vi "Loop Async.vi"(11 "RemoteDataService in":refnum<class "RemoteDataService.lvclass">) -> ()   [LabVIEW 2020, in "Vecto.lvlib" / "RemoteDataService.lvclass"]
uses:
  RemoteDataService.lvclass
  RemoteDataService.lvclass/RemoteDataService.ctl
  Packet.ctl
  lv-protoc/LV-Proto/Message/Message.lvclass
  Vecto.lvlib
  GroupNamesValue/GroupNamesValue.lvclass
  lv-promises/Promises/Promise/Promise.lvclass
  Group Data Type.ctl
  VectoConfig/VectoConfig.lvlib
  Publish Group Data.ctl
  EventLoggingService/EventLoggingService.lvclass
panel:
  out "Proc":i32(graph)
  out "Chart":i32(graph)
  out "Local Port":u16
  out "Bind Port":u16
  out "Bind Address":u32
  out "Node ID":u32
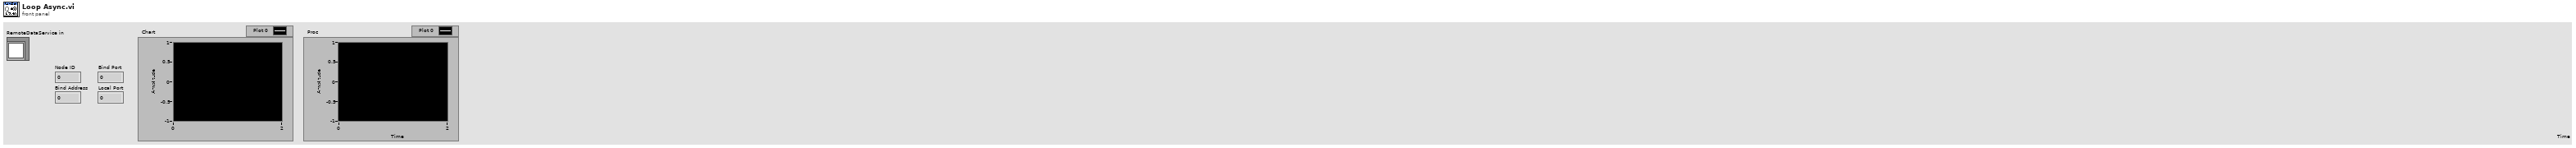
[diagram p1: front panel]
types:
  T1 = typedef "Vecto.lvlib/RemoteDataService.lvclass/Packet.ctl" = cluster{"UDP":refnum<k16>, "IP":u32, "Port":u16, "Message":refnum<class "Message.lvclass">, "Data Type":T2}
  T2 = typedef "VectoConfig.lvlib/Group Data Type.ctl" = enum16{"Double", "String", "Bool"}
  T3 = typedef "Vecto.lvlib/RemoteDataService.lvclass/Loop Data.ctl" = cluster{"Group Map":map{string, T4}, "UDP":refnum<k16>, "SequenceCountService":refnum<class "SequenceCountService.lvclass">, "Node ID":u32, "Bind Address":u32, "Bind Port":u16, "Local Port":u16, "TX Q":refnum<queue>, "Subscriptions":map{T5, T6}, "ChannelService":refnum<class "ChannelService.lvclass">, "Telemetry Config":T7}
  T4 = typedef "Vecto.lvlib/RemoteDataService.lvclass/Published Group.ctl" = cluster{"Last Publish":dbl, "Publish Address":u32, "Publish Port":u16}
  T5 = typedef "Vecto.lvlib/RemoteDataService.lvclass/Subscription.ctl" = cluster{"Multicast Address":string, "Multicast Port":u16}
  T6 = typedef "Vecto.lvlib/RemoteDataService.lvclass/Subscription Info.ctl" = cluster{"Close":refnum<user-event>, "New Data Handler":refnum<user-event>}
  T7 = typedef "VectoConfig.lvlib/Telemetry Config.ctl" = cluster{"Routing":T8, "Endpoint":T9}
  T8 = typedef "VectoConfig.lvlib/Telemetry Routing.ctl" = enum16{"Multicast", "Unicast"}
  T9 = typedef "VectoConfig.lvlib/Endpoint.ctl" = cluster{"Address":string, "Port":u16}
  T10 = typedef "Vecto.lvlib/RemoteDataService.lvclass/Publish Group Data.ctl" = cluster{"Data Msg":refnum<class "Message.lvclass">, "Group Name":string, "Data Type":T2}
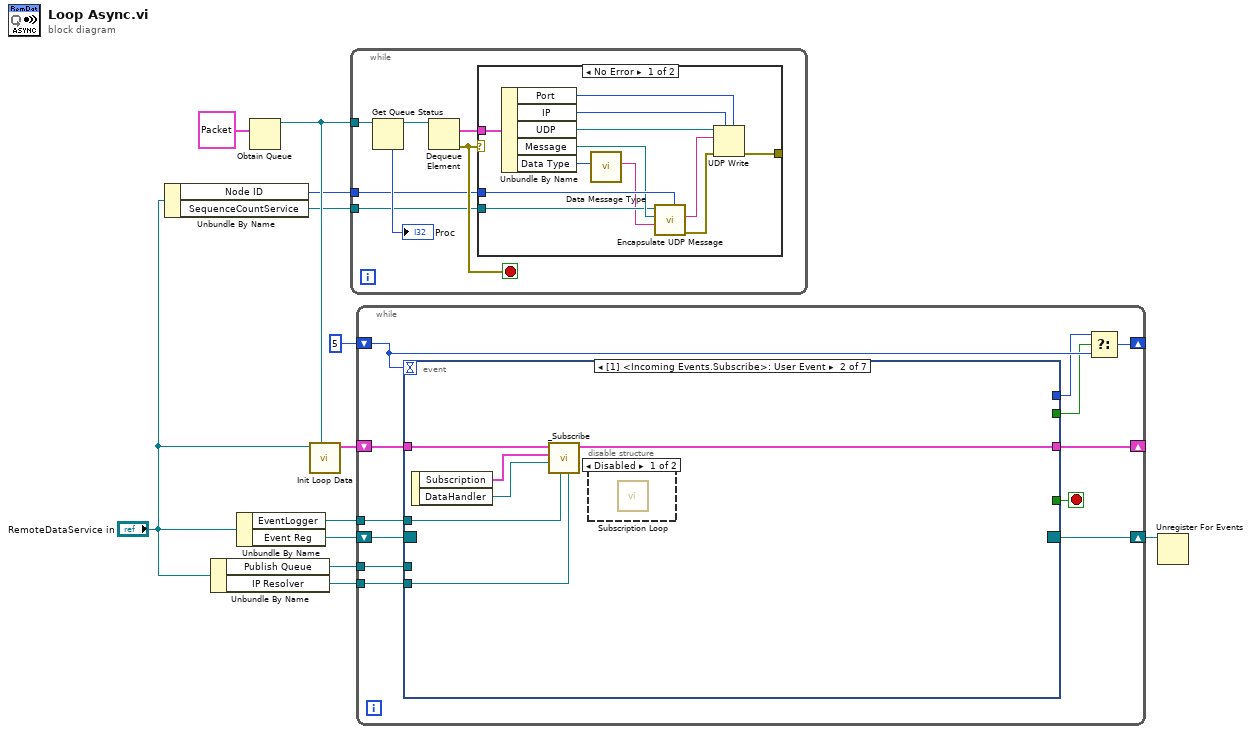
[diagram p0: block diagram]
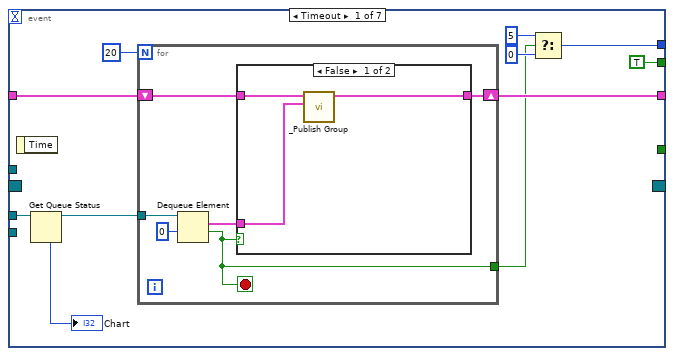
[diagram p3: hidden frame]
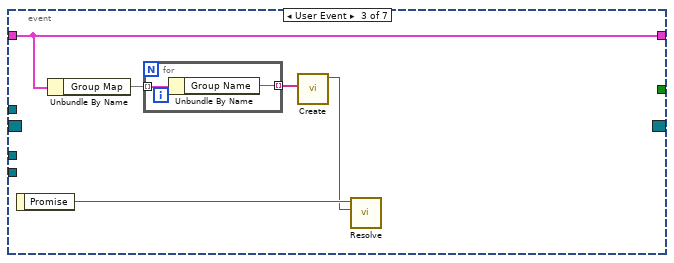
[diagram p6: hidden frame]
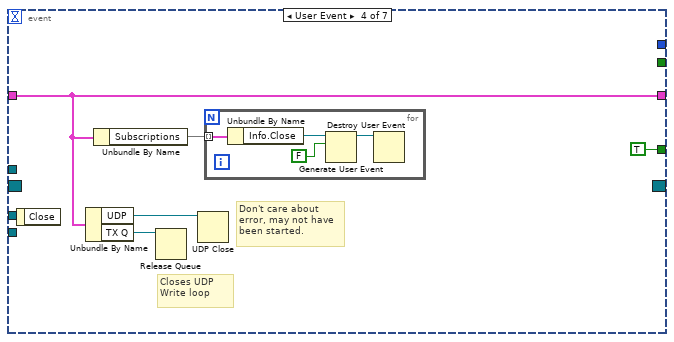
[diagram p7: hidden frame]
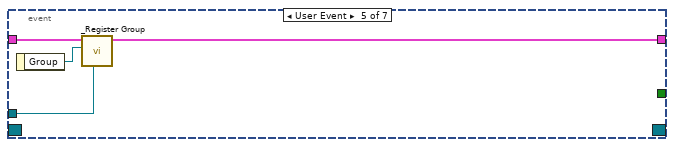
[diagram p8: hidden frame]
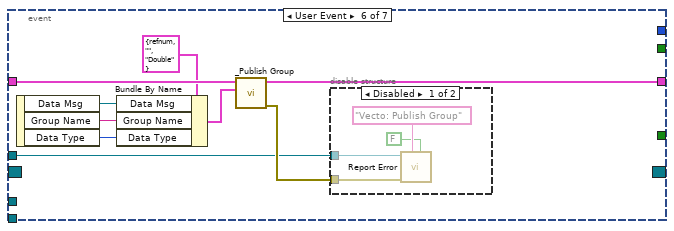
[diagram p9: hidden frame]
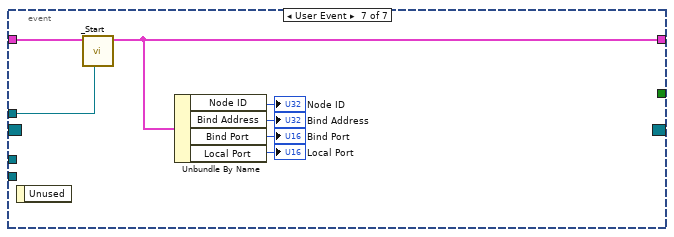
[diagram p11: hidden frame]
diagram:
  n1 = Unbundle By Name("RemoteDataService in") -> ("Node ID"=w5:u32, "SequenceCountService"=w4:refnum<class "SequenceCountService.lvclass">)
  n2 = Unbundle By Name("RemoteDataService in") -> ("Publish Queue"=w9:refnum<queue>, "IP Resolver"=w1:refnum<class "IP Resolver.lvclass">)
  n3 = Unbundle By Name("RemoteDataService in") -> ("EventLogger"=w2:refnum<class "EventLoggingService.lvclass">, "Event Reg"=w12:refnum<event-registration>)
  n4 = Obtain Queue(element data type=T1 {"UDP"=refnum, "IP"=0, "Port"=0, "Message"=refnum, "Data Type"=enum."Double"} ("Packet")) -> (queue out=w7:refnum<queue>)  [unwired: 4 in, 2 out]
  n5 = call "Init Loop Data.vi"("TX Q"=w7, "RemoteDataService in"="RemoteDataService in") -> ("Loop Data"=w10:T3)  [unwired: 8 in, 1 out]
  n6 = while {
    tunnel: w7 -> [w19]
    tunnel: w5 -> [w14]
    tunnel: w4 -> [w13]
    stop <- w17 stop-if-true
    n7 = Get Queue Status(queue=w19) -> (queue out=w16:refnum<queue>, # elements in queue=→"Proc":i32)  [unwired: 2 in, 6 out]
    n8 = Dequeue Element(queue=w16) -> (element=w18:T1, error out=w17:errorcluster)  [unwired: 2 in, 2 out]
    n9 = case shown="No Error" w17 {
      tunnel: w18 -> [w31 _]
      tunnel: w14 -> [w27 _]
      tunnel: w13 -> [w25 _]
      tunnel: [w20 _] -> _
      frame No Error {
        n10 = Unbundle By Name(w31) -> ("Port"=w28:u16, "IP"=w29:u32, "UDP"=w30:refnum<k16>, "Message"=w26:refnum<class "Message.lvclass">, "Data Type"=w22:T2)
        n11 = call "Data Message Type.vi"("Group Data Type"=w22) -> ("Message Type"=w21:string)  [unwired: 10 in]
        n12 = call "Encapsulate UDP Message.vi"("source_id"=w27, "type"=w21, "Encapsulated Msg"=w26, "SequenceCountService"=w25) -> ("error out"=w23:errorcluster, "UDP Payload"=w24:string)  [unwired: 6 in]
        n13 = UDP Write(address=w29, port or service name=w28, connection ID=w30, data in=w24, 8:w23) -> (error out=w20:errorcluster)  [unwired: 1 in, 1 out]
      }
      frame Error {
      }
    }
  }
  n14 = while {
    shift-right: [w41] -> w11
    shift-left: w12 -> [w43]
    shift-right: [w40] -> _
    shift-left: w10 -> [w42]
    tunnel: w9 -> [w38]
    shift-right: [w37] -> _
    shift-left: 5 -> [w36]
    tunnel: w2 -> [w33]
    tunnel: w1 -> [w32]
    stop <- w39 stop-if-true
    n15 = event shown="[1] <Incoming Events.Subscribe>: User Event" {
      selector: w43 -> [_ _ _ _ _ _ _]
      dyn-events: [_ _ _ _ _ _ _] -> w41
      timeout: w36 -> [_ _ _ _ _ _ _]
      tunnel: w42 -> [w51 w70 w75 w78 w90 w98 w110]
      tunnel: [w50 w69 w75 w78 w89 w97 w109] -> w40
      tunnel: [_ _ _ TRUE _ _ _] -> w39
      tunnel: w38 -> [w54 _ _ _ _ _ _]
      tunnel: [w45 _ _ _ _ _ _] -> w35
      tunnel: [TRUE _ _ _ _ _ _] -> w34
      tunnel: w33 -> [_ w67 _ _ w87 w91 w104]
      tunnel: w32 -> [_ w65 _ _ _ _ _]
      event Timeout {
        n16 = event-data() -> ()  [unwired: 1 in, 1 out]
        n17 = Get Queue Status(queue=w54) -> (queue out=w52:refnum<queue>, # elements in queue=→"Chart":i32)  [unwired: 2 in, 6 out]
        n18 = for {
          N: 20 -> [_]
          tunnel: w52 -> [w60]
          shift-right: [w56] -> w50
          shift-left: w51 -> [w57]
          tunnel: [w55] -> w46
          stop <- w55 stop-if-true
          n19 = Dequeue Element(queue=w60, timeout in ms (-1)=0) -> (element=w58:T10, timed out?=w55:bool)  [unwired: 1 in, 2 out]
          n20 = case shown="False" w55 {
            tunnel: w58 -> [w61 _]
            tunnel: w57 -> [w63 w64]
            tunnel: [w62 w64] -> w56
            frame False {
              n21 = call "_Publish Group.vi"("Publish Group Data"=w61, "Loop Data In"=w63) -> ("Loop Data"=w62:T3)  [unwired: 8 in, 1 out]
            }
            frame True {
            }
          }
        }
        n22 = Select(t=5, s=w46, f=0) -> (s? t:f=w45:i32)
      }
      event User Event {
        n23 = event-data() -> ("Subscription"=w68:T5, "DataHandler"=w66:refnum<class "SubscribedDataHandler.lvclass">)  [unwired: 1 in]
        n24 = call "_Subscribe.vi"("IP Resolver"=w65, "EventLogging"=w67, "DataHandler"=w66, "Subscription"=w68, "Loop Data In"=w70) -> ("Loop Data"=w69:T3)  [unwired: 5 in, 1 out]
        n25 = disable-structure shown="Disabled" {
          frame Disabled {
            n26 = call "Subscription Loop.vi"() -> ()  [unwired: 12 in]
          }
          frame Enabled {
          }
        }
      }
      event User Event {
        n27 = event-data() -> ("Promise"=w72:refnum<class "Promise.lvclass">)  [unwired: 1 in]
        n28 = Unbundle By Name(w75) -> ("Group Map"=w74:map{string, T4})
        n29 = for {
          tunnel: w74 -> [w77] mode=indexing
          tunnel: [w76] -> w73 mode=indexing
          n30 = Unbundle By Name(w77) -> ("Group Name"=w76:string)
        }
        n31 = call "Create.vi"("Groups"=w73) -> ("GroupsValue out"=w71:refnum<class "GroupNamesValue.lvclass">)  [unwired: 10 in]
        n32 = call "Resolve.vi"("Result (None)"=w71, "Promise in"=w72) -> ()  [unwired: 8 in, 2 out]
      }
      event User Event {
        # "Closes UDP Write loop"
        # "Don't care about error, may not have been started."
        n33 = event-data() -> ()  [unwired: 1 in, 1 out]
        n34 = Unbundle By Name(w78) -> ("UDP"=w81:refnum<k16>, "TX Q"=w80:refnum<queue>)
        n35 = Unbundle By Name(w78) -> ("Subscriptions"=w79:map{T5, T6})
        n36 = Release Queue(queue=w80) -> ()  [unwired: 2 in, 3 out]
        n37 = UDP Close(connection ID=w81) -> ()  [unwired: 1 in, 2 out]
        n38 = for {
          tunnel: w79 -> [w86] mode=indexing
          n39 = Unbundle By Name(w86) -> ("Info.Close"=w85:refnum<user-event>)
          n40 = Generate User Event(user event=w85, event data cluster=FALSE ("event data")) -> (user event out=w83:refnum<user-event>)  [unwired: 2 in, 1 out]
          n41 = Destroy User Event(user event=w83) -> ()  [unwired: 1 in, 1 out]
        }
      }
      event User Event {
        n42 = event-data() -> ("Group"=w88:refnum<class "Group.lvclass">)  [unwired: 1 in]
        n43 = call "_Register Group.vi"("EventLogging"=w87, "Group"=w88, "Loop Data In"=w90) -> ("Loop Data"=w89:T3)  [unwired: 7 in, 1 out]
      }
      event User Event {
        n44 = event-data() -> ("Data Msg"=w94:refnum<class "Message.lvclass">, "Group Name"=w93:string, "Data Type"=w92:T2)  [unwired: 1 in]
        n45 = Bundle By Name(cluster=T10 {"Data Msg"=refnum, "Group Name"="", "Data Type"=enum."Double"} ("Publish Group Data"), "Data Msg"=w94, "Group Name"=w93, "Data Type"=w92) -> (w95:T10)
        n46 = call "_Publish Group.vi"("Publish Group Data"=w95, "Loop Data In"=w98) -> ("error out"=w99:errorcluster, "Loop Data"=w97:T3)  [unwired: 8 in]
        n47 = disable-structure shown="Disabled" {
          disable-tunnel: w99 -> [w103 _]
          disable-tunnel: w91 -> [w102 _]
          frame Disabled {
            n48 = call "Report Error.vi"("Callchain (T)"=FALSE, "Context (None)"="Vecto: Publish Group", "error in (no error)"=w103, "EventLoggingService in"=w102) -> ()  [unwired: 6 in, 2 out]
          }
          frame Enabled {
          }
        }
      }
      event User Event {
        n49 = event-data() -> ()  [unwired: 1 in, 1 out]
        n50 = call "_Start.vi"("EventLogging"=w104, "Loop Data In"=w110) -> ("Loop Data"=w109:T3)  [unwired: 8 in, 1 out]
        n51 = Unbundle By Name(w109) -> ("Node ID"=→"Node ID":u32, "Bind Address"=→"Bind Address":u32, "Bind Port"=→"Bind Port":u16, "Local Port"=→"Local Port":u16)
      }
    }
    n52 = Select(t=w35, s=w34, f=w36) -> (s? t:f=w37:i32)
  }
  n53 = Unregister For Events(event registration refnum=w11) -> ()  [unwired: 1 in, 1 out]
